vi "RVHR - Configure Distance Slider.vi"(5 "Settings":T1, 6 "Local Data in":T3, 7 "UI Refs":T2, 8 "error in (no error)":errorcluster) -> (0 "error out":errorcluster, 4 "Local Data out":T3)   [LabVIEW 2024]
uses:
  Controls/RVHR - Local Data.ctl
  Controls/Test Cluster.ctl
  Controls/Excluded Information.ctl
  Controls/Language.ctl
  Controls/Device_Type.ctl
  <vilib>/Utility/miscctls.llb/LVRectTypeDef.ctl
  <vilib>/Utility/miscctls.llb/LVBoundsTypeDef.ctl
  Controls/RVHR - UI Refs.ctl
  Controls/RVHR - Reporting Settings.ctl
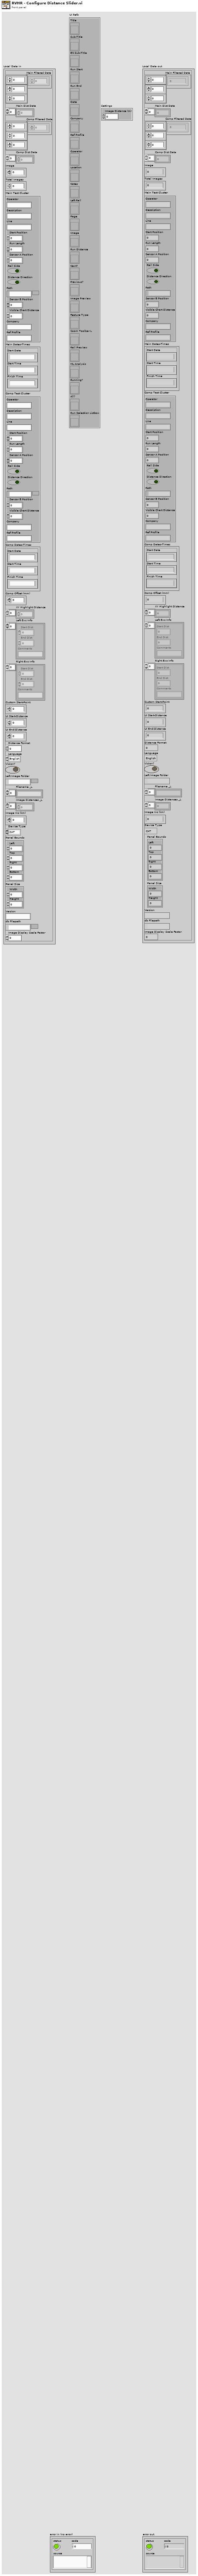
[diagram p1: front panel]
types:
  T1 = typedef "RVHR - Reporting Settings.ctl" = cluster{"Image Distance (m)":dbl}
  T2 = typedef "RVHR - UI Refs.ctl" = cluster{"Title":refnum<vi>, "Sub-Title":refnum<vi>, "EN Sub-Title":refnum<vi>, "Run Start":refnum<vi>, "Run End":refnum<vi>, "Date":refnum<vi>, "Company":refnum<vi>, "Ref Profile":refnum<vi>, "Operator":refnum<vi>, "Location":refnum<vi>, "Notes":refnum<vi>, "Left Rail":refnum<vi>, "Page":refnum<vi>, "Image":refnum<vi>, "Run Distance":refnum<vi>, "Next?":refnum<vi>, "Previous?":refnum<vi>, "Image Preview":refnum<vi>, "Feature Type:":refnum<vi>, "Zoom Toolbar L":refnum<vi>, "Rail Preview":refnum<vi>, "ML Analysis":refnum<vi>, "Running?":refnum<vi>, "All?":refnum<vi>, "Run Selection Listbox":refnum<vi>}
  T3 = typedef "RVHR - Local Data.ctl" = cluster{"Main Filtered Data":dbl[][][], "Main Dist Data":dbl[], "Comp Filtered Data":dbl[][][], "Comp Dist Data":dbl[], "Image":u16, "Total Images":u16, "Main Test Cluster":T4, "Main Dates-Times":cluster{"Start Date":string, "Start Time":string, "Finish Time":string}, "Comp Test Cluster":T4, "Comp Dates-Times":cluster{"Start Date":string, "Start Time":string, "Finish Time":string}, "Comp Offset (mm)":i64, "XY Highlight Distance":dbl[], "Left Exc Info":T5[], "Right Exc Info":T5[], "Custom Start-Point":dbl, "UI Start-Distance":dbl, "UI End-Distance":dbl, "Distance Format":u8, "Language":T6, "Vision?":bool, "Left Image Folder":path, "Filename _L":string[], "Image Distances _L":dbl[], "Image Inc (km)":dbl, "Device Type":T7, "Panel Bounds":T8, "Panel Size":T9, "Version":string, "db Filepath":path, "Image Display Scale Factor":dbl}
  T4 = typedef "Test Cluster.ctl" = cluster{"Operator":string, "Description":string, "Line":string, "Start Position":dbl, "Run Length":dbl, "Sensor A Position":dbl, "Rail Side":bool, "Distance Direction":bool, "Path":path, "Sensor B Position":dbl, "Visible Chart Distance":dbl, "Company":string, "Ref Profile":string}
  T5 = typedef "Excluded Information.ctl" = cluster{"Start Dist":dbl, "End Dist":dbl, "Comments":string}
  T6 = typedef "Language.ctl" = enum16{"English", "Chinese", "German"}
  T7 = typedef "Device_Type.ctl" = enum16{"CAT", "Bi-CAT", "YRCA", "RCA", "RV-HR", "TV-HR"}
  T8 = typedef "LVRectTypeDef.ctl" = cluster{"Left":i16, "Top":i16, "Right":i16, "Bottom":i16}
  T9 = typedef "LVBoundsTypeDef.ctl" = cluster{"Width":u32, "Height":u32}
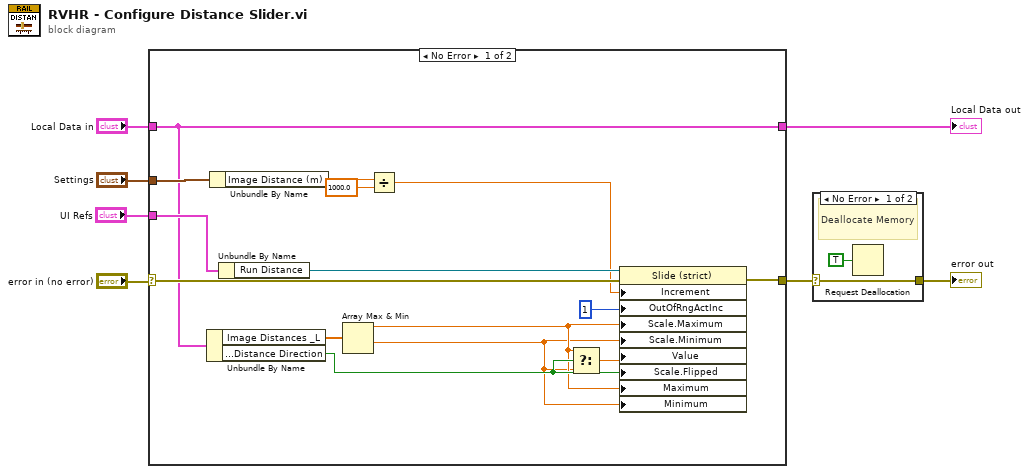
[diagram p0: block diagram]
diagram:
  n1 = case shown="No Error" "error in (no error)" {
    selector: "error in (no error)" -> [w21 w23]
    tunnel: "UI Refs" -> [w20 _]
    tunnel: [w15 w24] -> w5
    tunnel: "Local Data in" -> [w15 w24]
    tunnel: [w19 w23] -> w2
    tunnel: "Settings" -> [w18 _]
    frame No Error {
      n2 = Unbundle By Name(w15) -> ("Image Distances _L"=w13:dbl[], "Main Test Cluster.Distance Direction"=w10:bool)
      n3 = Unbundle By Name(w18) -> ("Image Distance (m)"=w17:dbl)
      n4 = Unbundle By Name(w20) -> ("Run Distance"=w22:refnum<vi>)
      n5 = Array Max & Min(array=w13) -> (max value=w9:dbl, min value=w8:dbl)  [unwired: 2 out]
      n6 = Divide(x=w17, y=1000.0) -> (x/y=w14:dbl)
      n7 = Select(t=w9, s=w10, f=w8) -> (s? t:f=w11:dbl)
      n8 = property class="Slide (strict)"(reference=w22, error in=w21, "Increment"=w14, "OutOfRngActInc"=u8 1 ("Response to Value Outside Limits:Increment"), "Scale.Maximum"=w9, "Scale.Minimum"=w8, "Value"=w11, "Scale.Flipped"=w10, "Maximum"=w9, "Minimum"=w8) -> (error out=w19:errorcluster)  [unwired: 1 out]
    }
    frame Error {
    }
  }
  "Local Data out" <- w5
  n9 = case shown="No Error" w2 {
    selector: w2 -> [w25 w27]
    tunnel: [w25 w27] -> w1
    frame No Error {
      # "Deallocate Memory"
      n10 = Request Deallocation(TRUE ("flag")) -> ()
    }
    frame Error {
    }
  }
  "error out" <- w1
